vi "Get Freq-RPM Spectral Map (U8).vi"(7 "dB On (T)":bool=TRUE, 8 "error in (no error)":errorcluster, 9 "Gabor template":dbl[](array[numeric]) format="%.2f", 10 "sampling frequency [Hz]":dbl=1.0 format="%.2f", 11 "RefNum in":T1) -> (0 "error out":errorcluster, 1 "quantization info":cluster{"offset":dbl, "multiplier":dbl} {"multiplier" format="%.2f"; "offset" format="%.2f"}, 2 "spectral map":u8[][](array[numeric]), 3 "RefNum out":T1, 4 "frequency scale":cluster{"offset":dbl, "multiplier":dbl} {"multiplier" format="%.2f"; "offset" format="%.2f"}, 5 "rpm scale":cluster{"offset":dbl, "multiplier":dbl} {"multiplier" format="%.2f"; "offset" format="%.2f"})   [LabVIEW 2017, in "SoundVib_Gabor.lvlib"]
doc: "Generates a frequency-rpm spectral map of the data block referenced by <B>RefNum in</B>. You can use this polymorphic VI to return <B>spectral map</B> as a 2D array of double-precision, floating-point numbers or a 2D array of 8-bit unsigned integers. You must manually select the polymorphic instance to use. Use the DBL instance to obtain more accurate data. Use the U8 instance to reduce memory usage when the VI displays data."
uses:
  <vilib>/addons/Sound and Vibration/Order Analysis/Gabor Order Tracking/SoundVib_Gabor.lvlib
  <vilib>/addons/Sound and Vibration/Order Analysis/Ref Gabor Order Tracking/GT RefNum.ctl
  <resource>/sndvib.dll
panel:
  # "Get Freq-RPM Spectral Map (U8)"
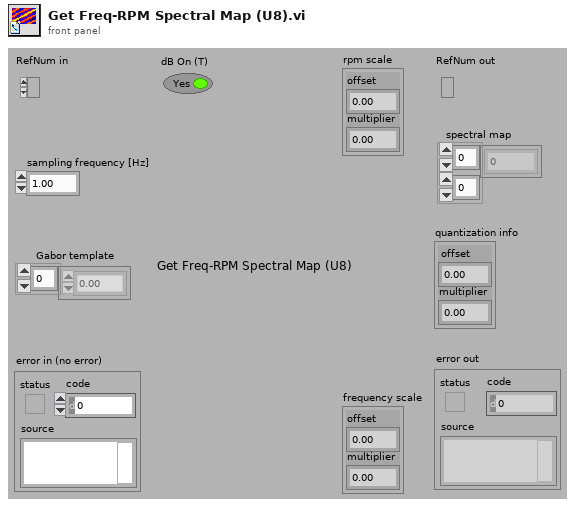
[diagram p1: front panel]
types:
  T1 = typedef "SoundVib_Gabor.lvlib/GT RefNum.ctl" = refnum<k1>
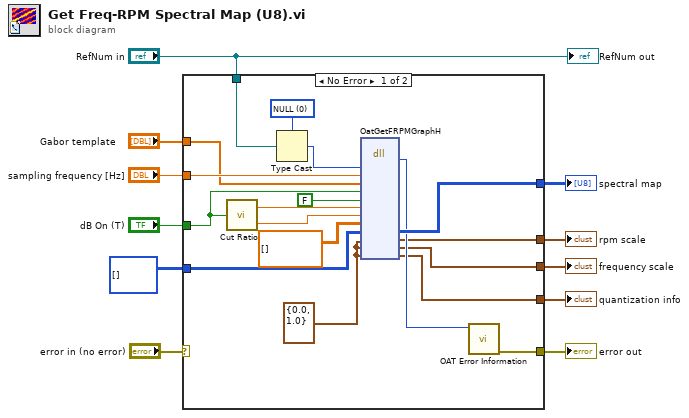
[diagram p0: block diagram]
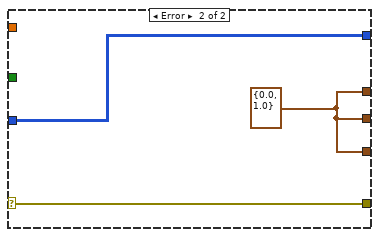
[diagram p2: hidden frame]
diagram:
  n1 = case shown="No Error" "error in (no error)" {
    selector: "error in (no error)" -> [_ w32]
    tunnel: [w29 w32] -> w6
    tunnel: "RefNum in" -> [w27 _]
    tunnel: [w12 w30] -> w9
    tunnel: [w16 w31] -> w10
    tunnel: [w14 w30] -> w2
    tunnel: "sampling frequency [Hz]" -> [w25 _]
    tunnel: "dB On (T)" -> [w23 _]
    tunnel: "Gabor template" -> [w24 _]
    tunnel: u8[][] [] ("Graph") -> [w21 w31]
    tunnel: [w13 w30] -> w1
    frame No Error {
      w22 = cluster{"Z Min":dbl, "Z Step":dbl} {"Z Min"=0.0, "Z Step"=1.0}
      w28 = u32 0 items=["NULL"]
      n2 = call <vilib>:"Cut Ratio.vi"("dB On (T)"=w23) -> ("UpperCutRatio"=w19:dbl, "LowerCutRatio"=w18:dbl)
      n3 = Type Cast(type=w28, x=w27) -> (*(type *) &x=w26:u32)
      n4 = dll-call lib="C:/Program Files (x86)/National Instruments/LabVIEW 2017/resource/sndvib.*" fn="OatGetFRPMGraphH"("Ref In"=w26, "fs"=w25, "CntFreq"=w24, "bLogZ"=w23, "bGetDBL"=FALSE ("dB On (T)"), "uCutRatio"=w19, "dCutRatio"=w18, "DBLGraph"=dbl[][] [], "U8Graph"=w21, "XScale"=w22, "YScale"=w22, "ZScale"=w22) -> ("return type"=w15:i32, "U8Graph"=w16:u8[][], "XScale"=w14:cluster{"Z Min":dbl, "Z Step":dbl}, "YScale"=w13:cluster{"Z Min":dbl, "Z Step":dbl}, "ZScale"=w12:cluster{"Z Min":dbl, "Z Step":dbl})  [unwired: 11 in, 2 out]
      n5 = call <vilib>:"OAT Error Information.vi"("error code"=w15) -> ("error out"=w29:errorcluster)  [unwired: 6 in]
    }
    frame Error {
      w30 = cluster{"Z Min":dbl, "Z Step":dbl} {"Z Min"=0.0, "Z Step"=1.0}
    }
  }
  "error out" <- w6
  "quantization info" <- w9
  "frequency scale" <- w1
  "rpm scale" <- w2
  "spectral map" <- w10
  "RefNum out" <- "RefNum in"
